vi "Change Conditional Disable Structure Value.vi"(7 "Project Path":path, 8 "error in (no error)":errorcluster, 10 "Requested Value":string="ON", 11 "Flag to find":string="DEBUG") -> (0 "error out":errorcluster, 2 "Array":cluster{"Symbol":string, "Value":string}[](array[cluster]))   [LabVIEW 2016]
doc: "Finds a conditional disable value in the current project and changes it to a requested value"
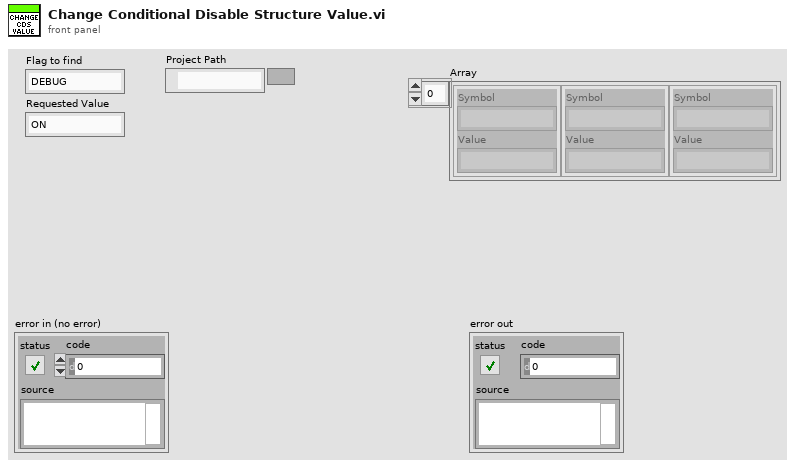
[diagram p1: front panel]
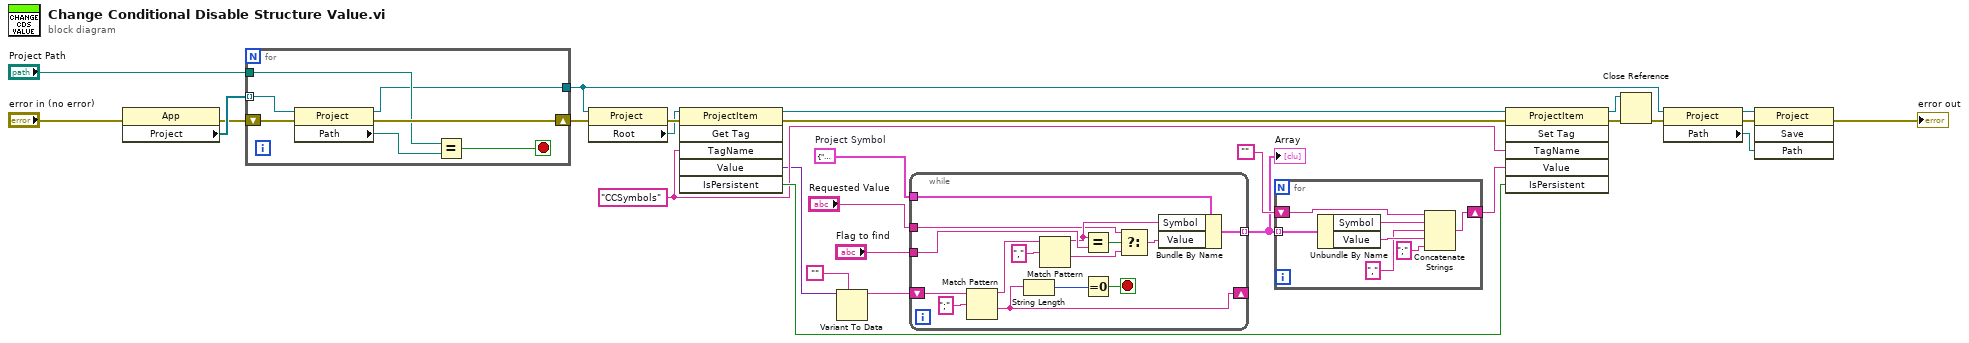
[diagram p0: block diagram]
diagram:
  w24 = cluster{"Symbol":string, "Value":string} {"Symbol"="", "Value"=""}  # Project Symbol
  w16 = "CCSymbols" ("Tag")
  n1 = property class="App"(error in="error in (no error)") -> (error out=w3:errorcluster, "Project"=w5:refnum<vi>[])  [unwired: 1 in, 1 out]
  n2 = for {
    tunnel: w5 -> [w35] mode=indexing
    tunnel: "Project Path" -> [w31]
    shift-right: [w32] -> w2
    shift-left: w3 -> [w33]
    tunnel: [w29] -> w1
    stop <- w30 stop-if-true
    n3 = property class="Project"(reference=w35, error in=w33) -> (reference out=w29:refnum<vi>, error out=w32:errorcluster, "Path"=w34:path)
    n4 = Equal?(x=w31, y=w34) -> (x = y?=w30:bool)
  }
  n5 = property class="Project"(reference=w1, error in=w2) -> (error out=w22:errorcluster, "Root"=w18:refnum<vi>)  [unwired: 1 out]
  n6 = invoke class="ProjectItem" method="Get Tag"(reference=w18, error in=w22, "TagName"=w16) -> (reference out=w15:refnum<vi>, error out=w21:errorcluster, "Value"=w13:variant, "IsPersistent"=w17:bool)  [unwired: 3 in, 2 out]
  n7 = Variant To Data(type="" ("Section"), Variant=w13) -> (data=w23:string)  [unwired: 1 in, 1 out]
  n8 = while {
    shift-right: [w48] -> _
    shift-left: w23 -> [w50]
    tunnel: w24 -> [w43]
    tunnel: [w42] -> w26 mode=indexing
    tunnel: "Flag to find" -> [w41]
    tunnel: "Requested Value" -> [w38]
    stop <- w46 stop-if-true
    n9 = Match Pattern(string=w50, regular expression=";") -> (before substring=w45:string, after substring=w48:string)  [unwired: 1 in, 2 out]
    n10 = String Length(string=w48) -> (length=w47:i32)
    n11 = Match Pattern(string=w45, regular expression=",") -> (before substring=w40:string, after substring=w37:string)  [unwired: 1 in, 2 out]
    n12 = Equal?(x=w40, y=w41) -> (x = y?=w39:bool)
    n13 = Equal To 0?(x=w47) -> (x = 0?=w46:bool)
    n14 = Select(t=w38, s=w39, f=w37) -> (s? t:f=w36:string)
    n15 = Bundle By Name(cluster=w43, "Symbol"=w40, "Value"=w36) -> (w42:cluster{"Symbol":string, "Value":string})
  }
  "Array" <- w26
  n16 = for {
    tunnel: w26 -> [w57] mode=indexing
    shift-right: [w56] -> w28
    shift-left: "" -> [w55]
    n17 = Unbundle By Name(w57) -> ("Symbol"=w54:string, "Value"=w53:string)
    n18 = Concatenate Strings(w55, w54, ",", w53, ";") -> (w56:string)
  }
  n19 = invoke class="ProjectItem" method="Set Tag"(reference=w15, error in=w21, "TagName"=w16, "Value"=w28, "IsPersistent"=w17) -> (reference out=w19:refnum<vi>, error out=w20:errorcluster)  [unwired: 1 in, 4 out]
  n20 = Close Reference(reference=w19, error in (no error)=w20) -> (error out=w7:errorcluster)
  n21 = property class="Project"(reference=w1, error in=w7) -> (reference out=w10:refnum<vi>, error out=w8:errorcluster, "Path"=w9:path)
  n22 = invoke class="Project" method="Save"(reference=w10, error in=w8, "Path"=w9) -> (error out=→"error out":errorcluster)  [unwired: 1 in, 3 out]
